vi "ClientGUIMonitorAllAnalog.vi"() -> ()   [LabVIEW 2021]
doc: "Le protocole UDP diffère du protocole TCP car il n'y a pas de détection d'erreur avec les paquets d'informations qui sont envoyés ; il n'y a donc aucune garantie qu'un destinataire reçoive bien des données.\n\nLe protocole UDP offre la possibilité de diffuser des données sur un réseau. Spécifiez simplement une adresse IP de uns (255.255.255.255) pour essayer de diffuser l'information sur tout le réseau. Gardez à l'esprit que des routeurs et d'autres périphériques de réseau refusent généralement de diffuser au-delà de certains points, la diffusion est donc limitée dans la pratique."
panel:
  out "Value":u16
  out "Pin11":cluster{string, bool, bool}[](graph)
  out "Pin10":cluster{string, bool, bool}[](graph)
  out "Pin9":cluster{string, bool, bool}[](graph)
  out "Pin8":cluster{string, bool, bool}[](graph)
  out "Pin7":cluster{string, bool, bool}[](graph)
  out "Pin6":cluster{string, bool, bool}[](graph)
  out "Value":u16
  out "Value":u16
  out "Value":u16
  out "Value":u16
  out "Value":u16
  out "Value":u16
  out "Value":u16
  out "Value":u16
  out "Value":u16
  out "Value":u16
  out "Value":bool
  in  "?":u32
  in  "Période\n(en ds)":u32(slide)=100 min=5 max=100 step=5 scale=5.0..100.0
  out "Pin5":cluster{string, bool, bool}[](graph)
  out "Pin4":cluster{string, bool, bool}[](graph)
  out "Pin3":cluster{string, bool, bool}[](graph)
  out "Pin2":cluster{string, bool, bool}[](graph)
  out "Pin1":cluster{string, bool, bool}[](graph)
  out "Pin0":cluster{string, bool, bool}[](graph)
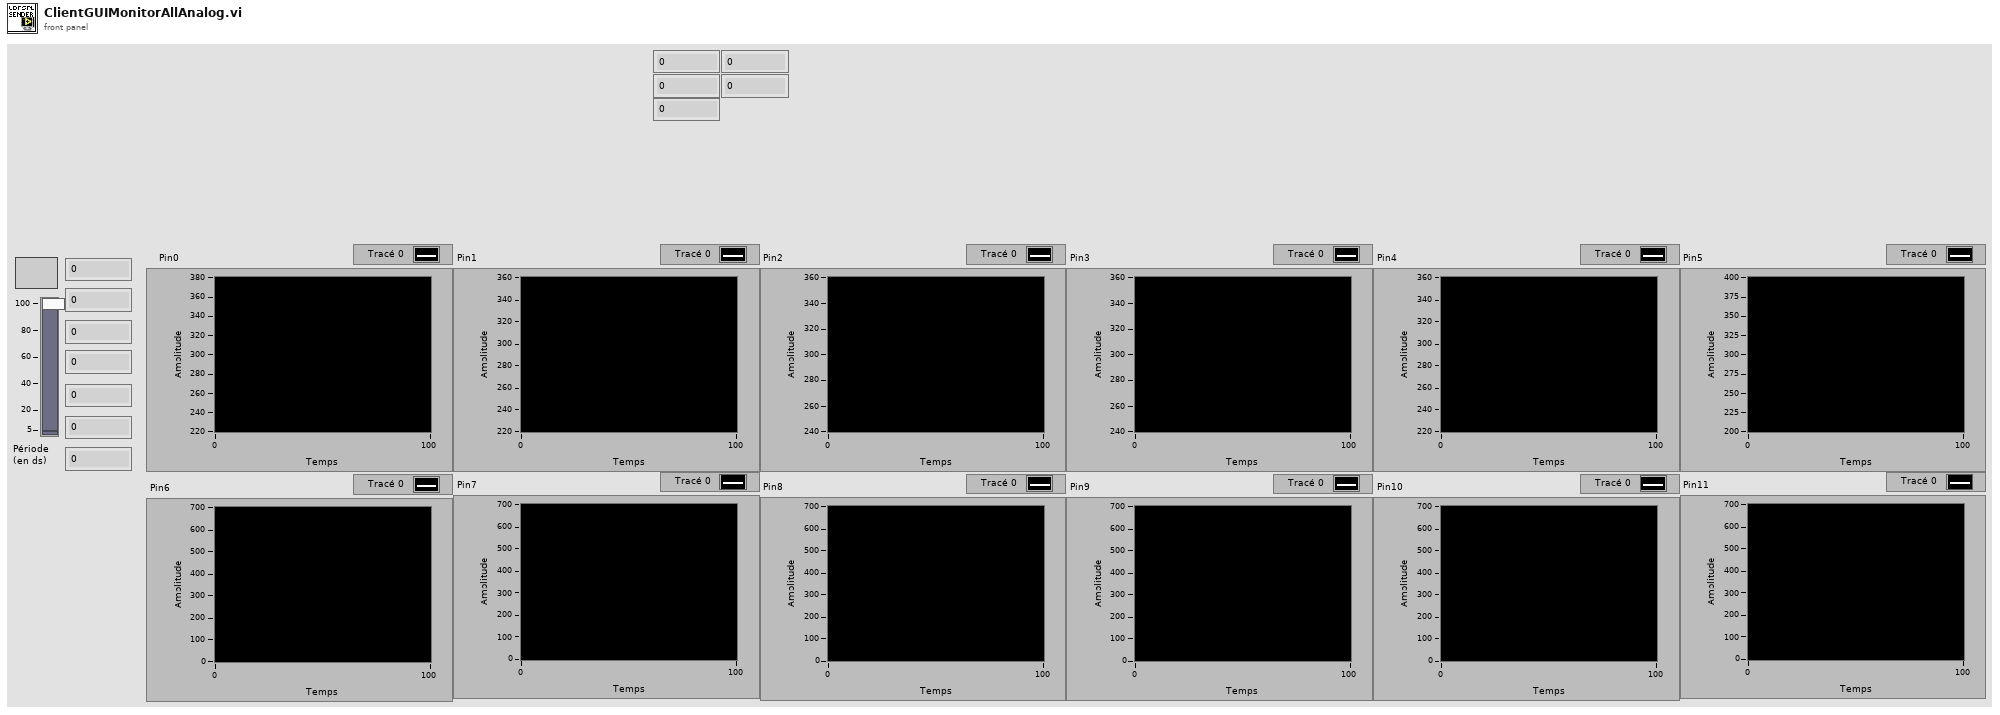
[diagram p1: front panel]
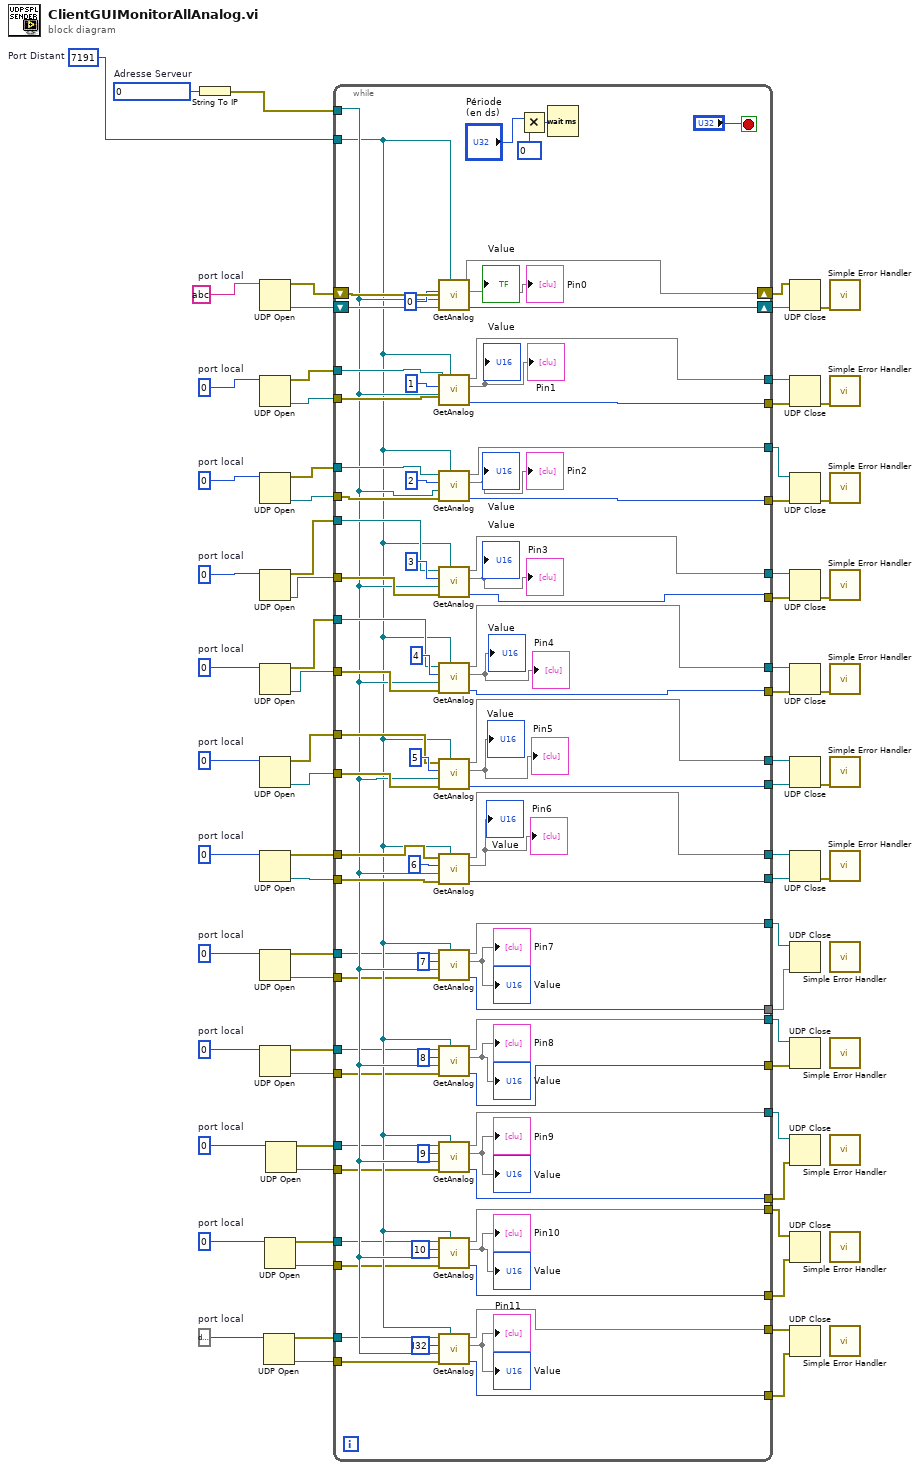
[diagram p0: block diagram]
diagram:
  w21 = data[3B]  # port local
  w22 = u16 0  # port local
  w23 = u16 0  # port local
  w24 = u16 0  # port local
  w25 = u16 0  # port local
  w56 = u16 0  # port local
  w57 = u16 0  # port local
  w58 = u16 0  # port local
  w59 = u16 0  # port local
  w60 = u16 0  # port local
  w61 = u16 0  # port local
  w68 = u16 7191  # Port Distant
  w67 = u16 0  # Adresse Serveur
  w70 = string data[3B]  # port local
  n1 = String To IP(1:w67) -> (0:w69:errorcluster)
  n2 = UDP Open(11:w70) -> (port=w66:errorcluster, 0:w65:refnum<k16>)  [unwired: 4 in, 1 out]
  n3 = UDP Open(11:w61) -> (port=w49:errorcluster, 0:w43:refnum<k16>)  [unwired: 4 in, 1 out]
  n4 = UDP Open(11:w60) -> (port=w48:errorcluster, 0:w42:refnum<k16>)  [unwired: 4 in, 1 out]
  n5 = UDP Open(11:w59) -> (port=w47:errorcluster, 0:w41:refnum<k16>)  [unwired: 4 in, 1 out]
  n6 = UDP Open(11:w58) -> (port=w46:errorcluster, 0:w40:refnum<k16>)  [unwired: 4 in, 1 out]
  n7 = UDP Open(11:w57) -> (port=w45:errorcluster, 0:w39:refnum<k16>)  [unwired: 4 in, 1 out]
  n8 = UDP Open(11:w56) -> (port=w44:errorcluster, 0:w38:refnum<k16>)  [unwired: 4 in, 1 out]
  n9 = UDP Open(11:w25) -> (port=w20:errorcluster, 0:w10:refnum<k16>)  [unwired: 4 in, 1 out]
  n10 = UDP Open(11:w24) -> (port=w19:errorcluster, 0:w9:refnum<k16>)  [unwired: 4 in, 1 out]
  n11 = UDP Open(11:w21) -> (port=w16:errorcluster, 0:w6:refnum<k16>)  [unwired: 4 in, 1 out]
  n12 = UDP Open(11:w22) -> (port=w17:errorcluster, 0:w7:refnum<k16>)  [unwired: 4 in, 1 out]
  n13 = UDP Open(11:w23) -> (port=w18:errorcluster, 0:w8:refnum<k16>)  [unwired: 4 in, 1 out]
  n14 = while {
    tunnel: w69 -> [w102]
    tunnel: w68 -> [w101]
    shift-right: [w103] -> w62
    shift-left: w66 -> [w145]
    shift-right: [w140] -> w63
    shift-left: w65 -> [w144]
    tunnel: w49 -> [w127]
    tunnel: w48 -> [w126]
    tunnel: w47 -> [w125]
    tunnel: w46 -> [w124]
    tunnel: w45 -> [w123]
    tunnel: w44 -> [w122]
    tunnel: w43 -> [w121]
    tunnel: w42 -> [w120]
    tunnel: w41 -> [w119]
    tunnel: w40 -> [w118]
    tunnel: w39 -> [w117]
    tunnel: w38 -> [w116]
    tunnel: [w115] -> w37
    tunnel: [w114] -> w36
    tunnel: [w113] -> w35
    tunnel: [w112] -> w34
    tunnel: [w111] -> w33
    tunnel: [w110] -> w32
    tunnel: [w109] -> w31
    tunnel: [w108] -> w30
    tunnel: [w107] -> w29
    tunnel: [w106] -> w28
    tunnel: [w105] -> w27
    tunnel: [w104] -> w26
    tunnel: w20 -> [w100]
    tunnel: w19 -> [w99]
    tunnel: w18 -> [w98]
    tunnel: w17 -> [w97]
    tunnel: w16 -> [w96]
    tunnel: [w90] -> w15
    tunnel: [w89] -> w14
    tunnel: [w88] -> w13
    tunnel: [w87] -> w12
    tunnel: [w86] -> w11
    tunnel: w10 -> [w85]
    tunnel: w9 -> [w84]
    tunnel: w8 -> [w83]
    tunnel: w7 -> [w82]
    tunnel: w6 -> [w81]
    tunnel: [w80] -> w5
    tunnel: [w79] -> w4
    tunnel: [w78] -> w3
    tunnel: [w77] -> w2
    tunnel: [w76] -> w1
    stop <- "?" stop-if-true
    n15 = call "GetAnalog.vi"(7:w101, 8:w144, 9:w102, 10:u8 0 ("Pin"), 11:w145) -> (0:w140:u16, 2:→"Pin0" →"Value", 3:w103)  [unwired: 4 in]
    n16 = call "GetAnalog.vi"(7:w101, 8:w121, 9:w102, 10:u8 1 ("Pin"), 11:w127) -> (0:w115:u16, 2:→"Pin1" →"Value", 3:w104)  [unwired: 4 in]
    n17 = call "GetAnalog.vi"(7:w101, 8:w120, 9:w102, 10:u8 2 ("Pin"), 11:w126) -> (0:w114:u16, 2:→"Pin2" →"Value", 3:w105)  [unwired: 4 in]
    n18 = call "GetAnalog.vi"(7:w101, 8:w119, 9:w102, 10:u8 3 ("Pin"), 11:w125) -> (0:w113:u16, 2:→"Pin3" →"Value", 3:w106)  [unwired: 4 in]
    n19 = call "GetAnalog.vi"(7:w101, 8:w118, 9:w102, 10:u8 4 ("Pin"), 11:w124) -> (0:w112:u16, 2:→"Pin4" →"Value", 3:w107)  [unwired: 4 in]
    n20 = call "GetAnalog.vi"(7:w101, 8:w117, 9:w102, 10:u8 5 ("Pin"), 11:w123) -> (0:w111:u16, 2:→"Pin5" →"Value", 3:w108)  [unwired: 4 in]
    n21 = call "GetAnalog.vi"(7:w101, 8:w116, 9:w102, 10:u8 6 ("Pin"), 11:w122) -> (0:w110:u16, 2:→"Pin6" →"Value", 3:w109)  [unwired: 4 in]
    n22 = call "GetAnalog.vi"(7:w101, 8:w85, 9:w102, 10:u8 7 ("Pin"), 11:w100) -> (0:w76:u16, 2:→"Pin7" →"Value", 3:w90)  [unwired: 4 in]
    n23 = call "GetAnalog.vi"(7:w101, 8:w84, 9:w102, 10:u8 8 ("Pin"), 11:w99) -> (0:w77:u16, 2:→"Pin8" →"Value", 3:w89)  [unwired: 4 in]
    n24 = call "GetAnalog.vi"(7:w101, 8:w83, 9:w102, 10:u8 9 ("Pin"), 11:w98) -> (0:w78:u16, 2:→"Pin9" →"Value", 3:w88)  [unwired: 4 in]
    n25 = call "GetAnalog.vi"(7:w101, 8:w82, 9:w102, 10:u8 10 ("Pin"), 11:w97) -> (0:w79:u16, 2:→"Pin10" →"Value", 3:w87)  [unwired: 4 in]
    n26 = call "GetAnalog.vi"(7:w101, 8:w81, 9:w102, 10:i32 u8 11 ("Pin"), 11:w96) -> (0:w80:u16, 2:→"Pin11" →"Value", 3:w86)  [unwired: 4 in]
    n27 = Multiply(x="Période\n(en ds)", y=u8 0) -> (x*y=w146:u32)
    n28 = Wait (ms)(milliseconds to wait=w146) -> ()  [unwired: 1 out]
  }
  n29 = UDP Close(connection ID=w62, 8:w63) -> (error out=w64:errorcluster)  [unwired: 1 out]
  n30 = UDP Close(connection ID=w26, 8:w37) -> (error out=w55:errorcluster)  [unwired: 1 out]
  n31 = UDP Close(connection ID=w27, 8:w36) -> (error out=w54:errorcluster)  [unwired: 1 out]
  n32 = UDP Close(connection ID=w28, 8:w35) -> (error out=w53:errorcluster)  [unwired: 1 out]
  n33 = UDP Close(connection ID=w29, 8:w34) -> (error out=w52:errorcluster)  [unwired: 1 out]
  n34 = UDP Close(connection ID=w30, 8:w33) -> (error out=w51:errorcluster)  [unwired: 1 out]
  n35 = UDP Close(connection ID=w31, 8:w32) -> (error out=w50:errorcluster)  [unwired: 1 out]
  n36 = UDP Close(connection ID=w15, 8:w1) -> ()  [unwired: 2 out]
  n37 = UDP Close(connection ID=w14, 8:w2) -> ()  [unwired: 2 out]
  n38 = UDP Close(connection ID=w13, 8:w3) -> ()  [unwired: 2 out]
  n39 = UDP Close(connection ID=w12, 8:w4) -> ()  [unwired: 2 out]
  n40 = UDP Close(connection ID=w11, 8:w5) -> ()  [unwired: 2 out]
  n41 = call <vilib>:"Simple Error Handler.vi"(9:w64) -> ()  [unwired: 4 in, 5 out]
  n42 = call <vilib>:"Simple Error Handler.vi"(9:w55) -> ()  [unwired: 4 in, 5 out]
  n43 = call <vilib>:"Simple Error Handler.vi"(9:w54) -> ()  [unwired: 4 in, 5 out]
  n44 = call <vilib>:"Simple Error Handler.vi"(9:w53) -> ()  [unwired: 4 in, 5 out]
  n45 = call <vilib>:"Simple Error Handler.vi"(9:w52) -> ()  [unwired: 4 in, 5 out]
  n46 = call <vilib>:"Simple Error Handler.vi"(9:w51) -> ()  [unwired: 4 in, 5 out]
  n47 = call <vilib>:"Simple Error Handler.vi"(9:w50) -> ()  [unwired: 4 in, 5 out]
  n48 = call <vilib>:"Simple Error Handler.vi"() -> ()  [unwired: 5 in, 5 out]
  n49 = call <vilib>:"Simple Error Handler.vi"() -> ()  [unwired: 5 in, 5 out]
  n50 = call <vilib>:"Simple Error Handler.vi"() -> ()  [unwired: 5 in, 5 out]
  n51 = call <vilib>:"Simple Error Handler.vi"() -> ()  [unwired: 5 in, 5 out]
  n52 = call <vilib>:"Simple Error Handler.vi"() -> ()  [unwired: 5 in, 5 out]
